vi "Communication.vi"(8 "Error In":errorcluster, 9 "Bytes to Read(I32)":i32, 10 "Command":string, 11 "connection ID":refnum<k5>) -> (0 "Error Out":errorcluster, 2 "Data out":string, 3 "connection ID out":refnum<k5>)   [LabVIEW 2019, in "FX5U SLMP Binary.lvlib"]
uses:
  FX5U SLMP Binary.lvlib
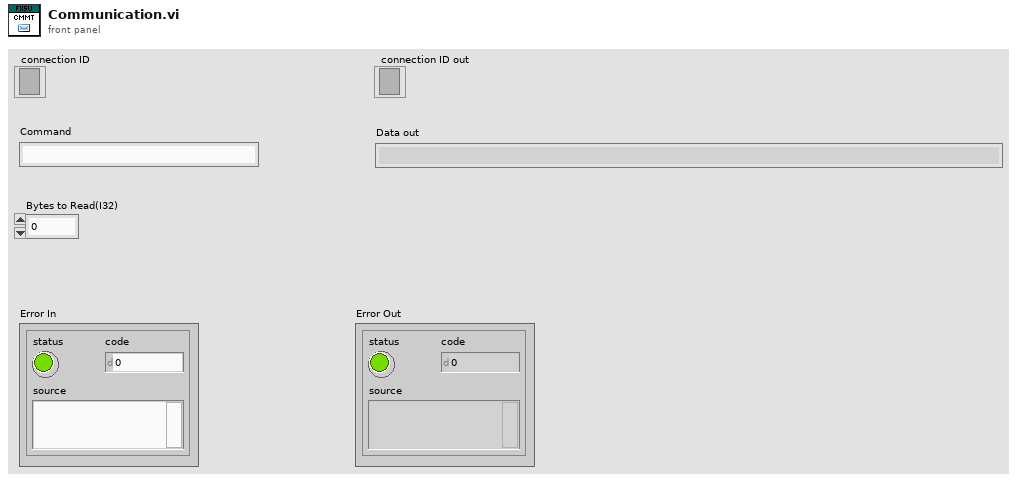
[diagram p1: front panel]
types:
  T1 = enum16{"big-endian, network order", "native, host order", "little-endian"}
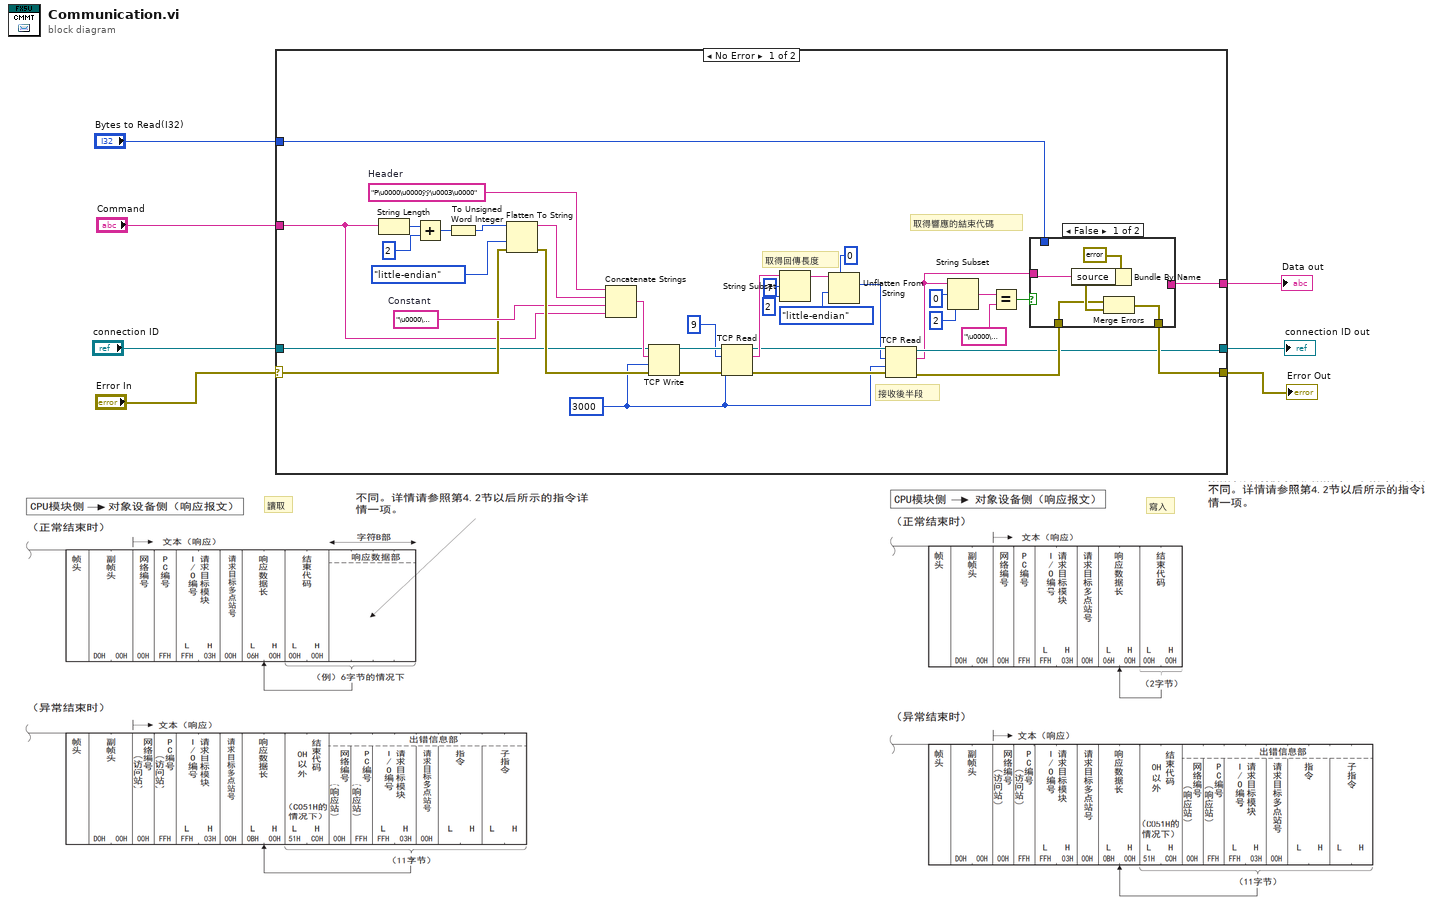
[diagram p0: block diagram]
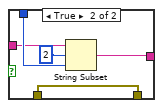
[diagram p2: hidden frame]
diagram:
  # "讀取"
  # "寫入"
  n1 = case shown="No Error" "Error In" {
    selector: "Error In" -> [w32 w55]
    tunnel: [w24 w55] -> w6
    tunnel: "connection ID" -> [w31 w56]
    tunnel: [w11 w56] -> w4
    tunnel: "Command" -> [w30 _]
    tunnel: "Bytes to Read(I32)" -> [w23 _]
    tunnel: [w22 _] -> w1
    frame No Error {
      w33 = "\u0000\u0000"  # Constant
      w41 = "P\u0000\u0000ÿÿ\u0003\u0000"  # Header
      w9 = 3000 ("timeout ms (25000)")
      # "接收後半段"
      # "取得回傳長度"
      # "取得響應的結束代碼"
      n2 = String Length(string=w30) -> (length=w40:i32)
      n3 = Add(x=w40, y=2) -> (x+y=w37:i32)
      n4 = To Unsigned Word Integer(number=w37) -> (unsigned 16bit integer=w38:u16)
      n5 = Flatten To String(anything=w38, byte order (0:big-endian, network order)=T1."little-endian", error in (no error)=w32) -> (data string=w35:string, error out=w34:errorcluster)  [unwired: 1 in, 1 out]
      n6 = Concatenate Strings(w41, w35, w33, w30) -> (w42:string)
      n7 = TCP Write(connection ID=w31, data in=w42, error in (no error)=w34, 9:w9) -> (connection ID out=w44:refnum<k5>, error out=w43:errorcluster)  [unwired: 1 out]
      n8 = TCP Read(connection ID=w44, bytes to read=9, error in (no error)=w43, 9:w9) -> (connection ID out=w13:refnum<k5>, data out=w18:string, error out=w14:errorcluster)  [unwired: 1 in]
      n9 = String Subset(string=w18, offset (0)=7, length (rest)=2 ("length (rest)")) -> (substring=w17:string)
      n10 = Unflatten From String(type=i16 0, binary string=w17, byte order (0:big-endian, network order)=T1."little-endian") -> (value=w10:i16)  [unwired: 2 in, 2 out]
      n11 = TCP Read(connection ID=w13, bytes to read=w10, error in (no error)=w14, 9:w9) -> (connection ID out=w11:refnum<k5>, data out=w8:string, error out=w12:errorcluster)  [unwired: 1 in]
      n12 = String Subset(string=w8, offset (0)=0, length (rest)=2 ("length (rest)")) -> (substring=w25:string)
      n13 = Equal?(x=w25, y="\u0000\u0000") -> (x = y?=w26:bool)
      n14 = case shown="False" w26 {
        tunnel: [w45 w51] -> w24
        tunnel: w8 -> [w47 w50]
        tunnel: w12 -> [w46 w51]
        tunnel: w23 -> [_ w54]
        tunnel: [_ w53] -> w22
        frame False {
          n15 = Bundle By Name(cluster=errorcluster {"status"=TRUE, "code"=0, "source"=""} ("error in (no error) 2"), "source"=w47) -> (w48:errorcluster)
          n16 = Merge Errors(w46, w48) -> (w45:errorcluster)
        }
        frame True {
          n17 = String Subset(string=w50, offset (0)=2, length (rest)=w54) -> (substring=w53:string)
        }
      }
    }
    frame Error {
    }
  }
  "Error Out" <- w6
  "connection ID out" <- w4
  "Data out" <- w1
